vi "WriteTagValue.vi"(8 "Number to Write":dbl, 9 "Value":string caption="Value to Write", 11 "Tag In":T2) -> ()   [LabVIEW 2016, in "Systemlink Tag.xctl"]
uses:
  Systemlink Tag.xctl
  SkylineCluster.ctl
  Systemlink Data.ctl
panel:
  out "Device In":T1={"Name"="", "BaseURL"="", "AppKey"="", "Headers"=["Content-Type:application/json"], "Timeout"=10000}
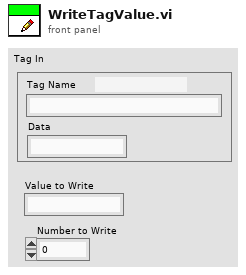
[diagram p1: front panel]
types:
  T1 = typedef "SkylineCluster.ctl" = cluster{"Name":string, "BaseURL":string, "AppKey":string, "Headers":string[], "Timeout":i32}
  T2 = typedef "Systemlink Tag.xctl/Systemlink Data.ctl" = cluster{"Tag Name":string, "Type":string, "Data":string}
  T3 = cluster{"timestamp":string, "value":cluster{"type":string, "value":string}}
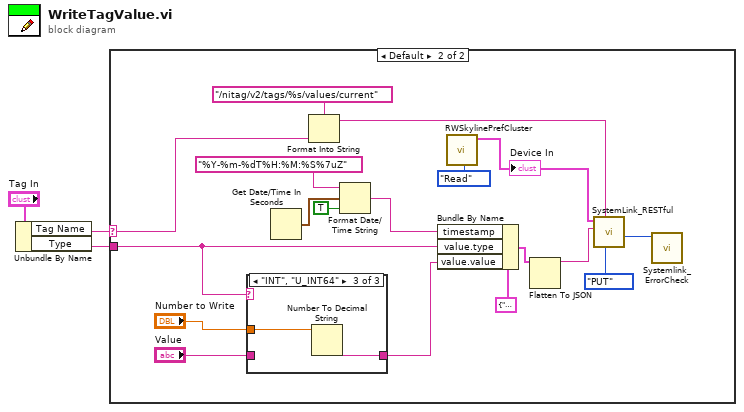
[diagram p0: block diagram]
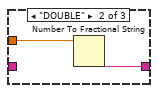
[diagram p4: hidden frame]
diagram:
  n1 = Unbundle By Name("Tag In") -> ("Tag Name"=w2:string, "Type"=w1:string)
  n2 = case shown="Default" w2 {
    selector: w2 -> [_ w13]
    tunnel: w1 -> [_ w7]
    frame "" {
    }
    frame Default {
      n3 = case shown="\"INT\", \"U_INT64\"" w7 {
        tunnel: "Number to Write" -> [_ w24 w26]
        tunnel: [w22 w23 w25] -> w8
        tunnel: "Value" -> [w22 _ _]
        frame Default {
        }
        frame "DOUBLE" {
          n4 = Number To Fractional String(number=w24) -> (F-format string=w23:string)  [unwired: 3 in]
        }
        frame "INT", "U_INT64" {
          n5 = Number To Decimal String(number=w26) -> (decimal integer string=w25:string)  [unwired: 1 in]
        }
      }
      n6 = Get Date/Time In Seconds() -> (seconds since 1Jan1904=w16:timestamp)
      n7 = Format Into String(format string="/nitag/v2/tags/%s/values/current" ("url"), w13) -> (resulting string=w21:string)  [unwired: 2 in, 1 out]
      n8 = Format Date/Time String(time format string (%c)="%Y-%m-%dT%H:%M:%S%7uZ", seconds (now)=w16, UTC format=TRUE) -> (date/time string=w18:string)
      n9 = Bundle By Name(cluster=T3 {"timestamp"="", "value"={"type"="", "value"=""}}, "timestamp"=w18, "value.type"=w7, "value.value"=w8) -> (w10:T3)
      n10 = call "RWSkylinePrefCluster.vi"("Task"=enum16{"Read", "Write"}."Read") -> ("Device Out"=w11:T1)  [unwired: 9 in, 1 out]
      "Device In" <- w11
      n11 = Flatten To JSON(anything=w10) -> (JSON string=w14:string)  [unwired: 2 in, 1 out]
      n12 = call "SystemLink_RESTful.vi"("Method"=enum16{"GET", "PUT", "POST", "MultiPOST"}."PUT", "url"=w21, "JSON"=w14, "Device In"=w11) -> ("HTTP Code"=w4:i32)  [unwired: 4 in, 3 out]
      n13 = call "Systemlink_ErrorCheck.vi"("HTTP Code"=w4) -> ()  [unwired: 11 in]
    }
  }
